vi "Set Cell (Timestamp).vi"(6 "Column":i32, 7 "Value":timestamp, 8 "error in (no error)":errorcluster, 9 "Row":i32, 10 "Sheet Reference":refnum<k24>) -> (0 "error out":errorcluster, 2 "Sheet Reference out":refnum<k24>)   [LabVIEW 2013]
uses:
  C:/PhaeronGit/LVNPOI/Resources/NPOI 2.1.1 dotnet2/NPOI.dll
  Resources/NPOI 2.1.1 dotnet2/NPOI.dll
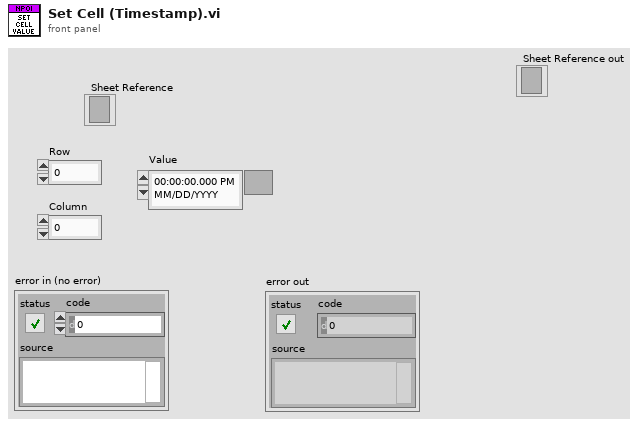
[diagram p1: front panel]
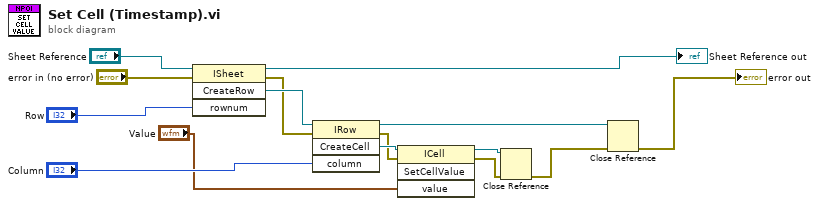
[diagram p0: block diagram]
diagram:
  n1 = invoke class="ISheet" method="CreateRow"(reference="Sheet Reference", error in="error in (no error)", "rownum"="Row") -> (reference out=→"Sheet Reference out":refnum<k24>, error out=w3:errorcluster, "CreateRow"=w12:refnum<k24>)  [unwired: 1 in, 1 out]
  n2 = invoke class="IRow" method="CreateCell"(reference=w12, error in=w3, "column"="Column") -> (reference out=w11:refnum<k24>, error out=w7:errorcluster, "CreateCell"=w8:refnum<k24>)  [unwired: 1 in, 1 out]
  n3 = invoke class="ICell" method="SetCellValue"(reference=w8, error in=w7, "value"="Value") -> (reference out=w6:refnum<k24>, error out=w5:errorcluster)  [unwired: 1 in, 2 out]
  n4 = Close Reference(reference=w6, error in (no error)=w5) -> (error out=w4:errorcluster)
  n5 = Close Reference(reference=w11, error in (no error)=w4) -> (error out=→"error out":errorcluster)
